vi "RF_Attn_init.vi"(1 "Initialize Instrument":u64, 2 "Inst_param":T1) -> ()   [LabVIEW 2013]
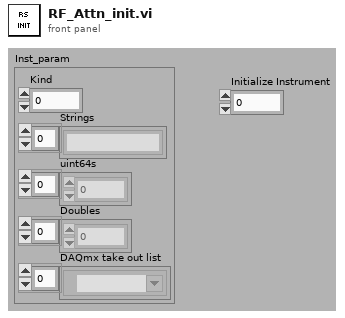
[diagram p1: front panel]
types:
  T1 = cluster{"Kind":u16, "Strings":string[], "uint64s":u64[], "Doubles":dbl[], "DAQmx take out list":refnum<k21>[]}
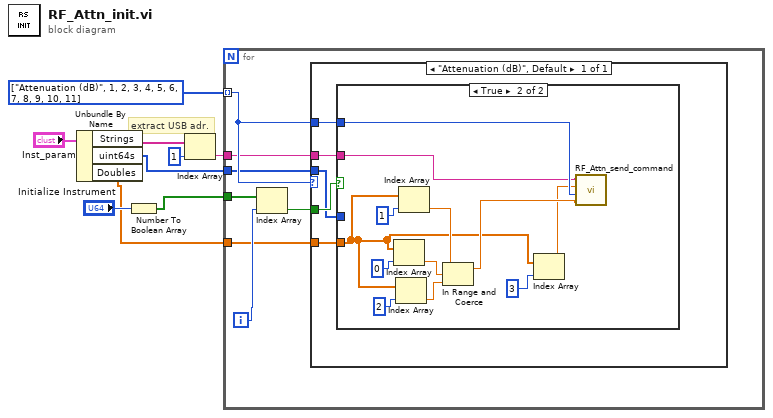
[diagram p0: block diagram]
diagram:
  w9 = enum16{"Attenuation (dB)"}[] [enum."Attenuation (dB)", 1, 2, 3, 4, 5, 6, 7, 8, 9, 10, 11] items=["Attenuation (dB)"]
  # "extract USB adr."
  n1 = Unbundle By Name("Inst_param") -> ("Strings"=w7:string[], "uint64s"=w2:u64[], "Doubles"=w1:dbl[])
  n2 = Number To Boolean Array(number="Initialize Instrument") -> (Boolean array=w3:bool[])
  n3 = Index Array(array=w7, index=1) -> (element=w5:string)
  n4 = for {
    tunnel: w9 -> [w14] mode=indexing
    tunnel: w5 -> [w12]
    tunnel: w3 -> [w16]
    tunnel: w2 -> [w11]
    tunnel: w1 -> [w10]
    i -> [w15]
    n5 = Index Array(array=w16, index=w15) -> (element=w13:bool)
    n6 = case shown="\"Attenuation (dB)\", Default" w14 {
      tunnel: w14 -> [w19]
      tunnel: w13 -> [w21]
      tunnel: w12 -> [w20]
      tunnel: w11 -> [w18]
      tunnel: w10 -> [w17]
      frame "Attenuation (dB)", Default {
        n7 = case shown="True" w21 {
          tunnel: w20 -> [_ w26]
          tunnel: w19 -> [_ w27]
          tunnel: w18 -> [_ _]
          tunnel: w17 -> [_ w23]
          frame False {
          }
          frame True {
            n8 = Index Array(array=w23, index=0) -> (element=w30:dbl)
            n9 = Index Array(array=w23, index=2) -> (element=w28:dbl)
            n10 = Index Array(array=w23, index=1) -> (element=w29:dbl)
            n11 = In Range and Coerce(upper limit=w29, x=w30, lower limit=w28) -> (coerced(x)=w25:dbl)  [unwired: 1 out]
            n12 = Index Array(array=w23, index=3) -> (element=w22:dbl)
            n13 = call "RF_Attn_send_command.vi"("Value"=w25, "Parameter"=w27, "Insertion Loss"=w22, "USB address"=w26) -> ()  [unwired: 1 in]
          }
        }
      }
    }
  }
